vi "Extract Step Number from TransID.vi"(10 "TransID":string="trans2011619111444.320[6 0 4]") -> (2 "Step":string)   [LabVIEW 2009]
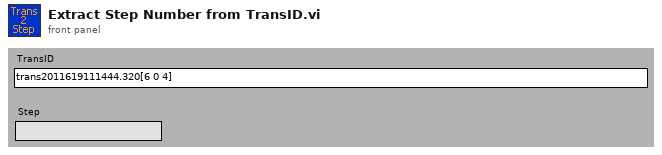
[diagram p1: front panel]
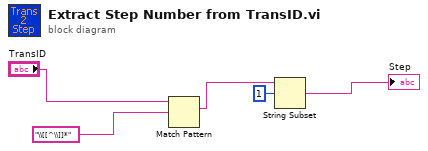
[diagram p0: block diagram]
diagram:
  n1 = Match Pattern(string="TransID", regular expression="\\[[^\\]]*") -> (match substring=w3:string)  [unwired: 1 in, 3 out]
  n2 = String Subset(string=w3, offset (0)=1) -> (substring=→"Step":string)  [unwired: 1 in]
